vi "M03 Hybrid Car.vi"(11 "EV3 in":T1) -> (3 "EV3 out":T1)   [LabVIEW 2016]
uses:
  <vilib>/NXT/Subs/LVHSConnector.ctl
  <vilib>/NXT/LegoClasses/BrickReference/BrickReference.lvclass
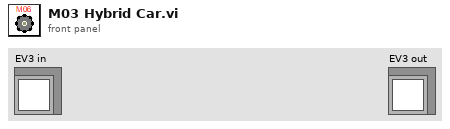
[diagram p1: front panel]
types:
  T1 = typedef "LVHSConnector.ctl" = refnum<class "BrickReference.lvclass">
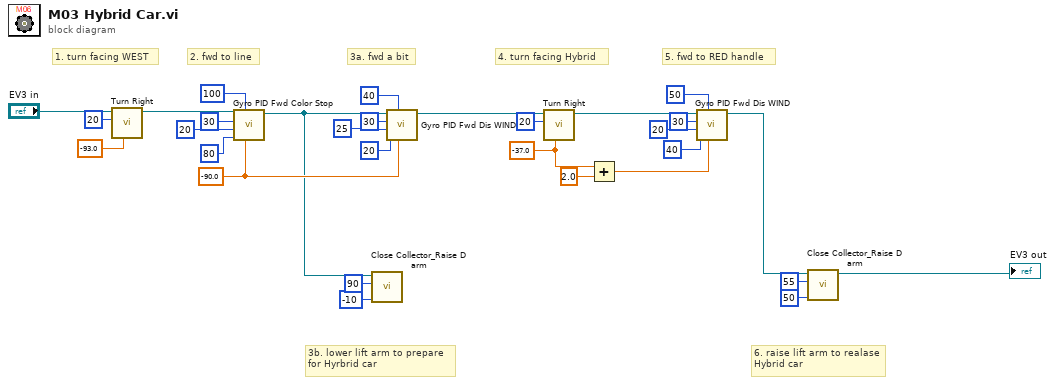
[diagram p0: block diagram]
diagram:
  w10 = sgl -37.0 ("Turning angle")
  w11 = sgl -90.0 ("Target angle")
  # "5. fwd to RED handle"
  # "4. turn facing Hybrid"
  # "3a. fwd a bit"
  # "2. fwd to line"
  # "1. turn facing WEST"
  # "3b. lower lift arm to prepare\nfor Hyrbrid car"
  # "6. raise lift arm to realase\nHybrid car"
  n1 = call "Turn Right.vi"("Turning angle"=sgl -93.0, "Motor B (right)"=i8 20, "EV3 in"="EV3 in") -> ("EV3 out"=w27:T1)  [unwired: 8 in]
  n2 = call "Gyro PID Fwd Color Stop.vi"("Target angle"=w11, "Threshold to Color"=100, "Threshold to slow"=80, "Min. speed"=20, "Max. speed"=30, "EV3 in"=w27) -> ("EV3 out"=w5:T1)  [unwired: 5 in]
  n3 = call "Close Collector_Raise D arm.vi"("Power"=i8 -10, "Rotation"=90, "EV3 in"=w5) -> ()  [unwired: 8 in, 1 out]
  n4 = call "Gyro PID Fwd Dis WIND.vi"("Target angle"=w11, "Threshold to stop"=40 ("Stop rotation"), "Threshold to slow"=20 ("Threshold to De-acc"), "Higher speed"=25 ("De-acc"), "Max. speed"=30 ("Acc"), "EV3 in"=w5) -> ("EV3 out"=w17:T1)  [unwired: 5 in]
  n5 = call "Turn Right.vi"("Turning angle"=w10, "Motor B (right)"=i8 20, "EV3 in"=w17) -> ("EV3 out"=w14:T1)  [unwired: 8 in]
  n6 = Add(x=w10, y=sgl 2.0) -> (x+y=w8:sgl)
  n7 = call "Gyro PID Fwd Dis WIND.vi"("Target angle"=w8, "Threshold to stop"=50 ("Stop rotation"), "Threshold to slow"=40 ("Threshold to De-acc"), "Higher speed"=20, "Max. speed"=30 ("Acc"), "EV3 in"=w14) -> ("EV3 out"=w2:T1)  [unwired: 5 in]
  n8 = call "Close Collector_Raise D arm.vi"("Power"=i8 50, "Rotation"=55, "EV3 in"=w2) -> ("EV3 out"=→"EV3 out":T1)  [unwired: 8 in]
